vi "Reset Handshake - Slave.vi"(0 "reset done":bool, 1 "reset handshake item":refnum<k21>) -> (4 "reset":bool)   [LabVIEW 2018, in "Streaming FPGA.lvlib"]
doc: "Creates the reset signal for the slave clock domain in a master-slave clock domain configuration.\n\nA true on the <B>reset</B> output signals a reset request (this output is set to true for one clock cycle). A true on the <B>reset done</B> input signals that the reset cycle is complete (this input is ignored if the <B>reset</B> output is true). The master clock domain must use the <B>Reset Handshake - Master</B> VI to process the reset requests and to create its own reset request signal. The reset signal for the master clock domain is already set to true by the time this VI sets its <B>reset</B> output to true, and the reset signal for the master clock domain remains true until the <B>reset done</B> input of this VI is false.\n\nThe resource wired to the <B>reset handshake item</B> input must be created by the <B>Reset Handshake - Create Resource</B> VI and this same resource must be wired to the <B><B>Reset Handshake - Master</B> VI as well."
uses:
  Streaming FPGA.lvlib
  <instrlib>/_niInstr/Basic Elements/v1/FPGA/Public/Max Fanout.ctl
  <vilib>/rvi/DataTransferAndStorage/Container/Common/niFpgaContainerExecOnDevCompGetState.vi
  <vilib>/rvi/Emulation/niFpgaEmulationIsFPGAContextNoSignature.vi
  <vilib>/rvi/DataTransferAndStorage/Container/Common/niFpgaContainerGetUniqueNameForEmu.vi
  <vilib>/rvi/eio/common/nirviEmuReportErrorAndStop.vi
  <vilib>/rvi/Emulation/niFpgaSctlEmulationGetInTimedLoop.vi
  <vilib>/rvi/Emulation/niFpgaProcessEmulError.vi
  <vilib>/rvi/DataTransferAndStorage/Container/XNode/niFpgaContainer.xnode
  <vilib>/rvi/DataTransferAndStorage/Handshake/Emulation/niFpgaHandshakeEmulationRefIn.vi
  <instrlib>/_niInstr/Basic Elements/v1/FPGA/niInstr Basic Elements v1 FPGA.lvlib
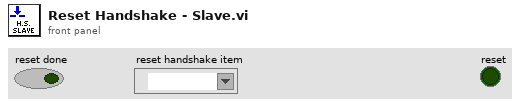
[diagram p1: front panel]
types:
  T1 = typedef "niInstr Basic Elements v1 FPGA.lvlib/Max Fanout.ctl" = enum16{"4", "8", "16", "32"}
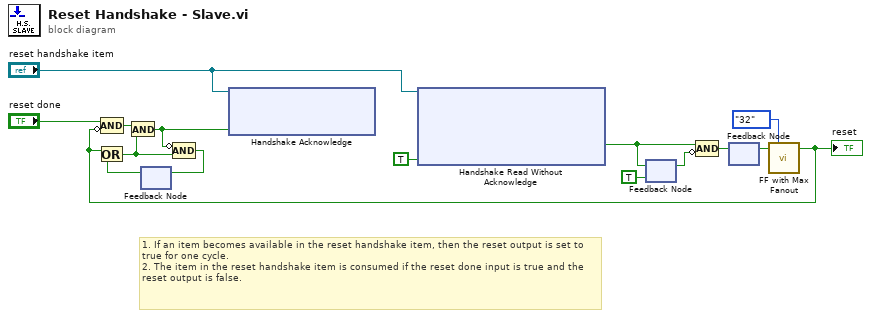
[diagram p0: block diagram]
diagram:
  # "1. If an item becomes available in the reset handshake item, then the reset output is set to true for one cycle.\n2. The item in the reset handshake item is consumed if the reset done input is true and the reset output is false."
  n1 = feedback #1() -> (w8:bool)  [unwired: 1 in]
  n2 = xnode "Handshake Read Without Acknowledge"("Ready for Output"=TRUE, "Handshake In"="reset handshake item") -> ("Output Valid"=w12:bool)  [unwired: 2 out]
  n3 = feedback-in #2(w12) -> ()
  n4 = feedback #2(TRUE ("Output Valid")) -> (w11:bool)
  n5 = Compound Arithmetic op=AND(w12, invert w11) -> (w2:bool)
  n6 = feedback #3() -> (w1:bool)  [unwired: 1 in]
  n7 = feedback-in #3(w2) -> ()
  n8 = call <instrlib>:"FF with Max Fanout.vi"("cDataIn"=w1, "kMaxFanout"=Max_Fanout."32") -> ("cDataOut"=w4:bool)  [unwired: 13 in]
  "reset" <- w4
  n9 = Or(x=w4, y=w8) -> (x .or. y?=w6:bool)
  n10 = Compound Arithmetic op=AND("reset done", invert w4) -> (w9:bool)
  n11 = And(x=w9, y=w6) -> (x .and. y?=w5:bool)
  n12 = Compound Arithmetic op=AND(invert w5, w6) -> (w7:bool)
  n13 = feedback-in #1(w7) -> ()
  n14 = xnode "Handshake Acknowledge"("Enable"=w5, "Handshake In"="reset handshake item") -> ()  [unwired: 1 out]
